vi "Lesker Serial read.vi"(6 "Number of reads":i32=1 min=1, 7 "VISA resource name":refnum<visa-resource-name>="COM7", 8 "error in (no error)":errorcluster, 10 "Serial Settings":T1={"baud rate"=19200, "data bits"=8, "parity"=enum."None", "stop bits"=10, "flow control"=0} {"flow control" items=["None"=0, "XON/XOFF"=1, "RTS/CTS"=2, "DTR/DSR"=4]; "stop bits" items=["1.0"=10, "1.5"=15, "2.0"=20]; "data bits" min=5 max=8 step=1; "baud rate" items=["75"=75, "110"=110, "134"=134, "150"=150, "300"=300, "600"=600, "1200"=1200, "1800"=1800, "2400"=2400, "4800"=4800, "7200"=7200, "9600"=9600, "14400"=14400, "19200"=19200, "28800"=28800, "38400"=38400, "56000"=56000, "57600"=57600, "115200"=115200, "128000"=128000, "230400"=230400]}, 11 "Command":string="#01RD") -> (0 "error out":errorcluster, 2 "Pressure":dbl=0.000289 format="%#_6e", 3 "Response":string="*01 2.89E-04\r")   [LabVIEW 2022 SP3]
doc: "This example performs a serial port write and a serial port read. The parameters set for the serial port must match the parameters of the connected instrument or device. The VISA Configure Serial Port VI sets the configuration parameters. The front panel displays the controls used to configure the basic parameters, such as baud rate, data bits, and parity. The VI passes the VISA resource name to other VIs that perform operations on that VISA resource. The VISA Write function sends a command to the serial device and the VISA Read function returns data based on the command. The VISA Close function then closes the reference to the serial device. It is important to close the reference; otherwise, further communication through that port might not be possible."
uses:
  Serial - Settings.ctl
  <vilib>/Analysis/baseanly.llb/Mean (DBL).vi
  <vilib>/Instr/_visa.llb/VISA Configure Serial Port (Instr).vi
  <vilib>/Analysis/NI_AALBase.lvlib
panel:
  out "##":i32
  out "bytes read":u32=13
  in  "delay before read (ms)":u32=50
  # "Overview: Demonstrates the use of the VISA functions to send a single command to a serial instrument and read a response.\nRequirements: NI-VISA Driver\nInstructions:\n1. Ensure the resource specified by the VISA resource name is a valid serial device.\n2. Run the VI.\n3. If your instrument recognizes the \"*IDN?\" command, it should return a Response."
  # "Note: For an example of how to perform continuous serial communication in a loop, open the Continuous Serial Write and Read.vi in the same folder as this example."
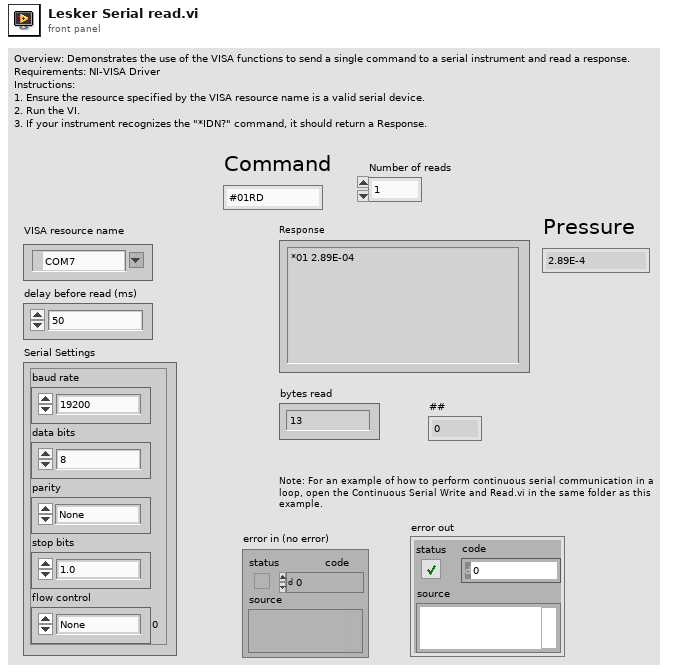
[diagram p1: front panel]
types:
  T1 = typedef "Serial - Settings.ctl" = cluster{"baud rate":u32, "data bits":u16, "parity":enum16{"None", "Odd", "Even", "Mark", "Space"}, "stop bits":u16, "flow control":u16}
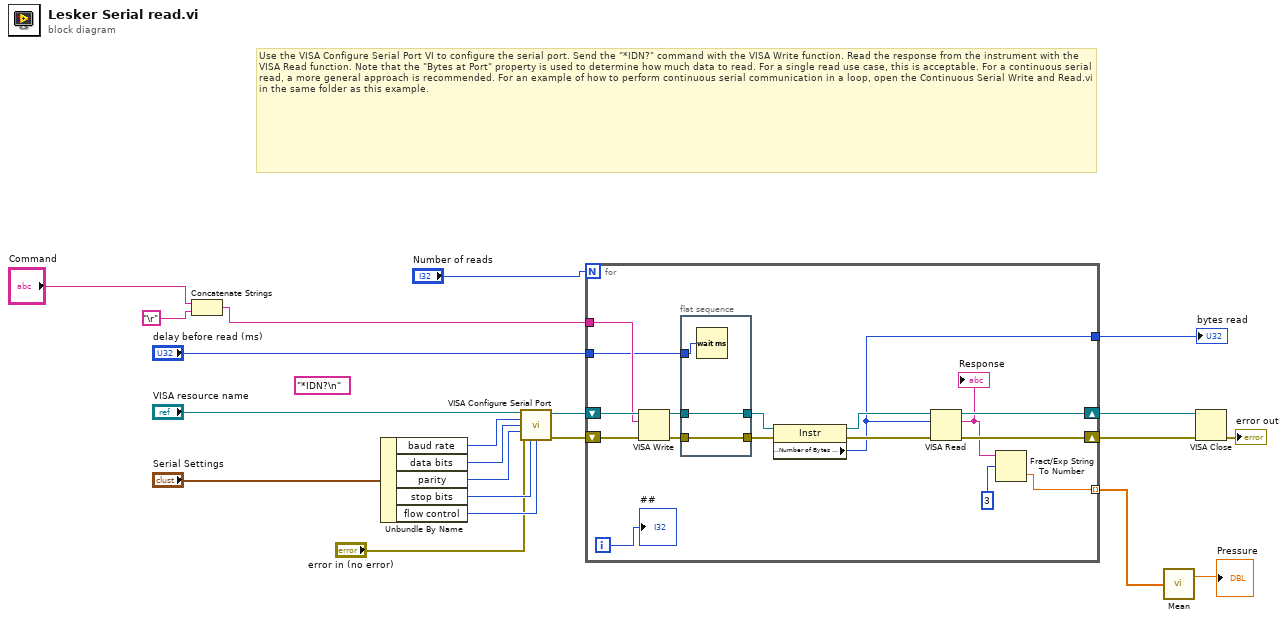
[diagram p0: block diagram]
diagram:
  (unwired) "*IDN?\n" ("Command")
  # "Use the VISA Configure Serial Port VI to configure the serial port. Send the \"*IDN?\" command with the VISA Write function. Read the response from the instrument with the VISA Read function. Note that the \"Bytes at Port\" property is used to determine how much data to read. For a single read use case, this is acceptable. For a continuous serial read, a more general approach is recommended. For an example of how to perform continuous serial communication in a loop, open the Continuous Serial Write and Read.vi in the same folder as this example."
  n1 = Concatenate Strings("Command", "\r") -> (w7:string)
  n2 = Unbundle By Name("Serial Settings") -> ("baud rate"=w14:u32, "data bits"=w13:u16, "parity"=w12:enum16{"None", "Odd", "Even", "Mark", "Space"}, "stop bits"=w11:u16, "flow control"=w10:u16)
  n3 = call-poly "VISA Configure Serial Port"("VISA resource name"="VISA resource name", "baud rate (9600)"=w14, "data bits (8)"=w13, "parity (0:none)"=w12, "error in (no error)"="error in (no error)", "stop bits (10: 1 bit)"=w11, "flow control (0:none)"=w10) -> ("VISA resource name out"=w19:refnum<visa-resource-name>, "error out"=w20:errorcluster)  [unwired: 2 in, 5 out]
  n4 = for {
    N: "Number of reads" -> [_]
    tunnel: [w28] -> w16
    tunnel: w7 -> [w27]
    tunnel: "delay before read (ms)" -> [w26]
    shift-right: [w36] -> w18
    shift-left: w20 -> [w38]
    shift-right: [w35] -> w17
    shift-left: w19 -> [w37]
    tunnel: [w23] -> w3 mode=indexing
    i -> [w22]
    n5 = VISA Write(VISA resource name=w37, write buffer=w27, error in (no error)=w38) -> (VISA resource name out=w32:refnum<visa-resource-name>, error out=w34:errorcluster)  [unwired: 1 out]
    n6 = flat-sequence {
      tunnel: w34 -> [w41]
      tunnel: [w41] -> w33
      tunnel: w32 -> [w40]
      tunnel: [w40] -> w31
      tunnel: w26 -> [w39]
      frame #0 {
        n7 = Wait (ms)(milliseconds to wait=w39) -> ()  [unwired: 1 out]
      }
    }
    n8 = property class="Instr"(reference=w31, error in=w33) -> (reference out=w30:refnum<visa-resource-name>, error out=w29:errorcluster, "Serial Settings:Number of Bytes at Serial Port"=w28:u32)
    n9 = VISA Read(VISA resource name=w30, byte count=w28, error in (no error)=w29) -> (VISA resource name out=w35:refnum<visa-resource-name>, read buffer=w24:string, error out=w36:errorcluster)  [unwired: 1 out]
    "Response" <- w24
    n10 = Fract/Exp String To Number(string=w24, offset=3) -> (number=w23:dbl)  [unwired: 2 in, 1 out]
    "##" <- w22
  }
  "bytes read" <- w16
  n11 = call-poly <vilib>:"Mean.vi"("X"=w3) -> ("mean"=→"Pressure":dbl)  [unwired: 1 out]
  n12 = VISA Close(VISA resource name=w17, error in (no error)=w18) -> (error out=→"error out":errorcluster)
